vi "read_attributes.vi"(8 "error in (no error)":errorcluster caption="entrée d'erreur (pas d'erreur)", 11 "DictionaryLearning en entrée":refnum<class "DictionaryLearning.lvclass">) -> (0 "error out":errorcluster caption="sortie d'erreur", 2 "attributes":T1, 3 "DictionaryLearning en sortie":refnum<class "DictionaryLearning.lvclass">)   [LabVIEW 2020, in "DictionaryLearning.lvclass"]
uses:
  DictionaryLearning.lvclass
  Controls/dictionary_learning_attributes.ctl
  DictionaryLearning.lvclass/DictionaryLearning.ctl
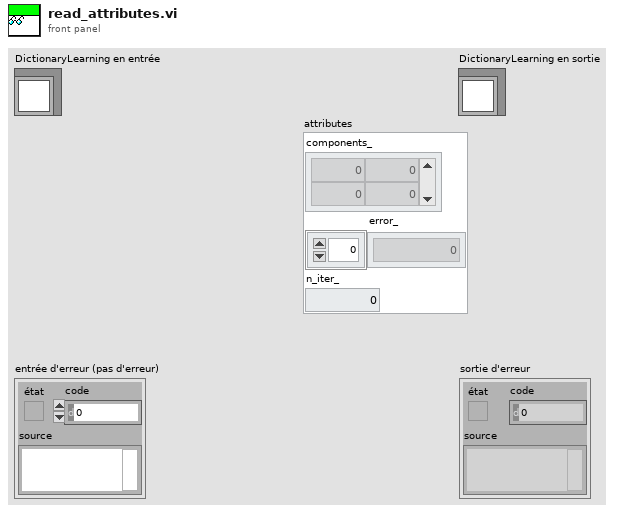
[diagram p1: front panel]
types:
  T1 = typedef "dictionary_learning_attributes.ctl" = cluster{"components_":dbl[][], "error_":dbl[], "n_iter_":dbl}
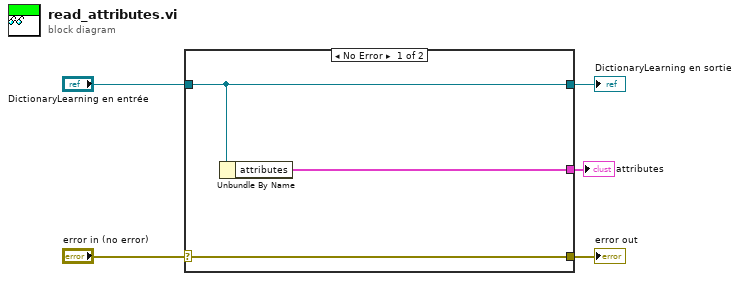
[diagram p0: block diagram]
diagram:
  n1 = case shown="No Error" "error in (no error)" {
    selector: "error in (no error)" -> [w8 w9]
    tunnel: [w8 w9] -> w4
    tunnel: [w7 w10] -> w2
    tunnel: "DictionaryLearning en entrée" -> [w7 w10]
    tunnel: [w6 _] -> w1
    frame No Error {
      n2 = Unbundle By Name(w7) -> ("attributes"=w6:T1)
    }
    frame Error {
    }
  }
  "error out" <- w4
  "DictionaryLearning en sortie" <- w2
  "attributes" <- w1
